vi "TDMS Advanced Asynchronous Write.vi"   [LabVIEW 2023]
doc: "This example demonstrates how to write data asynchronously to a .tdms file using the Advanced TDMS VIs and functions. You can use the TDMS Advanced Asynchronous Read function to read the data from the .tdms file."
panel:
  # "Overview: Demonstrates how to write data asynchronously to a .tdms file using the Advanced TDMS VIs and functions.\nInstructions:\nRun the VI."
types:
  T1 = enum16{"open", "open or create", "create or replace", "create", "open (read-only)"}
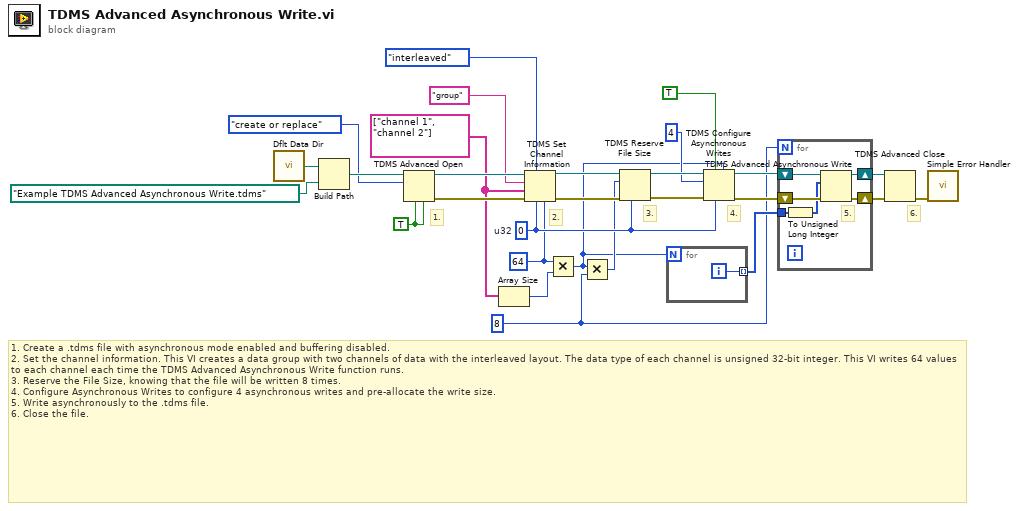
[diagram p0: block diagram]
diagram:
  w15 = TRUE ("enable asynchronous? (T)")
  w2 = 8 ("y")
  w4 = u32 64 ("samples per channel")
  w9 = u32 0  # u32
  w5 = string[] ["channel 1", "channel 2"] ("channel name(s)")
  # "4."
  # "1. Create a .tdms file with asynchronous mode enabled and buffering disabled.\n2. Set the channel information. This VI creates a data group with two channels of data with the interleaved layout. The data type of each channel is unsigned 32-bit integer. This VI writes 64 values to each channel each time the TDMS Advanced Asynchronous Write function runs.\n3. Reserve the File Size, knowing that the file will be written 8 times.\n4. Configure Asynchronous Writes to configure 4 asynchronous writes and pre-allocate the write size.\n5. Write asynchronously to the .tdms file.\n6. Close the file."
  # "1."
  # "6."
  # "3."
  # "2."
  n1 = call <vilib>:"Dflt Data Dir.vi"() -> ("App:Default Data Directory"=w23:path)
  n2 = Build Path(base path=w23, name or relative path=path "Example TDMS Advanced Asynchronous Write.tdms") -> (appended path=w27:path)
  n3 = TDMS Advanced Open(4:w15, 6:w15, 10:T1."create or replace" ("operation (0:open)"), 11:w27) -> (0:w25:errorcluster, 3:w24:refnum<k34>)  [unwired: 1 in, 1 out]
  n4 = Array Size(array=w5) -> (size(s)=w3:i32)
  n5 = TDMS Set Channel Information(4:w4, 6:w9, 7:enum16{"non-interleaved", "interleaved"}."interleaved" ("data layout (0:non-interleaved)"), 8:w25, 9:w5, 10:"group" ("group name (Untitled)"), 11:w24) -> (0:w17:errorcluster, 3:w16:refnum<k34>)
  n6 = Multiply(x=w4, y=w3) -> (x*y=w1:u32)
  n7 = Multiply(x=w1, y=w2) -> (x*y=w6:u32)
  n8 = TDMS Reserve File Size(6:w9, 8:w17, 10:w6, 11:w16) -> (0:w14:errorcluster, 3:w13:refnum<k34>)  [unwired: 1 in]
  n9 = for {
    N: w1 -> [_]
    tunnel: [w29] -> w20 mode=indexing
    i -> [w29]
  }
  n10 = TDMS Configure Asynchronous Writes(5:w1, 6:w9, 7:TRUE ("pre-allocate? (F)"), 8:w14, 10:u32 4 ("number of buffers (4)"), 11:w13) -> (0:w11:errorcluster, 3:w12:refnum<k34>)  [unwired: 1 in]
  n11 = for {
    N: w2 -> [_]
    shift-right: [w32] -> w18
    shift-left: w12 -> [w34]
    shift-right: [w33] -> w19
    shift-left: w11 -> [w35]
    tunnel: w20 -> [w31]
    # "5."
    n12 = To Unsigned Long Integer(number=w31) -> (unsigned 32bit integer=w30:u32[])
    n13 = TDMS Advanced Asynchronous Write(8:w35, 10:w30, 11:w34) -> (0:w33:errorcluster, 3:w32:refnum<k34>)
  }
  n14 = TDMS Advanced Close(8:w19, 11:w18) -> (0:w7:errorcluster)  [unwired: 2 in, 1 out]
  n15 = call <vilib>:"Simple Error Handler.vi"("error in (no error)"=w7) -> ()  [unwired: 4 in, 5 out]
